vi "HandleResponse.vi"(8 "error in (no error)":errorcluster, 10 "response":T1, 11 "BaseDriver in":refnum<class "BaseDriver.lvclass">) -> (0 "error out":errorcluster, 2 "Response out":T1[](array[typedef]), 3 "BaseDriver out":refnum<class "BaseDriver.lvclass">)   [LabVIEW 2025, in "BaseDriver.lvclass"]
doc: "Callback for any responses retreived from the remote destination. Overload this method to do any special handling in your driver"
uses:
  BaseDriver.lvclass
  response.ctl
  driver_status.ctl
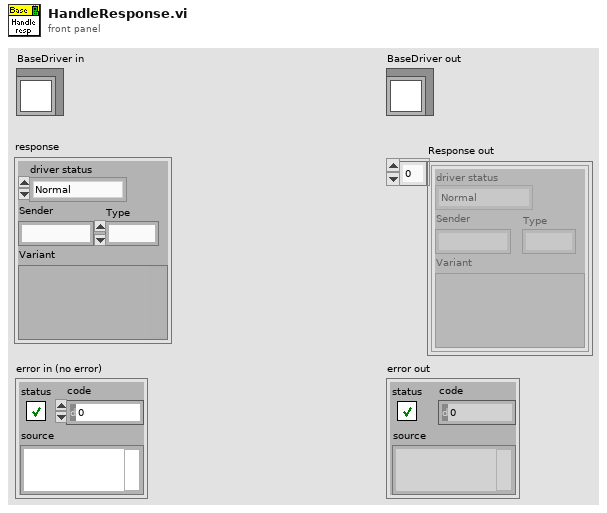
[diagram p1: front panel]
types:
  T1 = typedef "response.ctl" = cluster{"driver status":T2, "Sender":string, "Type":i32, "Variant":variant}
  T2 = typedef "driver_status.ctl" = enum16{"Normal", "Startup", "Connection lost", "Reconnected", "Timeout", "Idle", "Busy"}
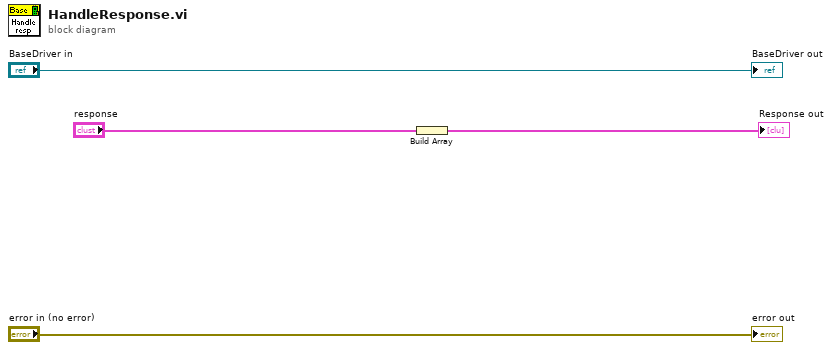
[diagram p0: block diagram]
diagram:
  n1 = Build Array("response") -> (→"Response out":T1[])
  "error out" <- "error in (no error)"
  "BaseDriver out" <- "BaseDriver in"
